vi "Laser Messenger.vi"(0 "Notifier Name":string, 2 "Action":T4, 5 "Emission On/Off":bool, 7 "Power (mW)":dbl, 11 "Laser Settings":T1, 13 "Exit While Busy (F)?":bool) -> (4 "Notifier Name Dup":string, 6 "Enabled (Interlock)?":bool, 8 "Light Emission?":bool, 10 "Laser Status":T3, 14 "Power (mW)":dbl, 15 "Laser Settings":T1)   [LabVIEW 2020]
uses:
  Laser Controls/Laser Actions.ctl
  Laser Controls/Laser Settings.ctl
  Laser Controls/Laser Parameters.ctl
  Laser Controls/Laser Status.ctl
  Laser Controls/Laser Notifier Element.ctl
panel:
  out "Error":errorcluster
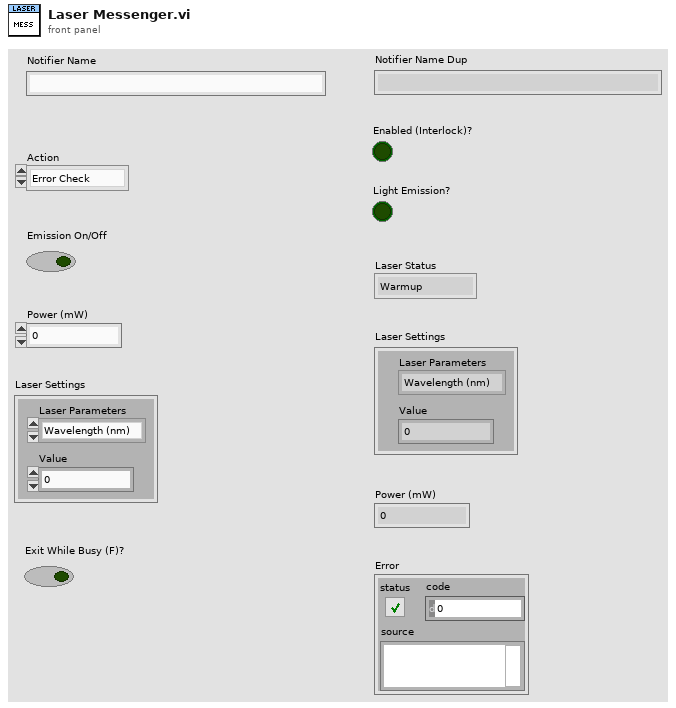
[diagram p1: front panel]
types:
  T1 = typedef "Laser Settings.ctl" = cluster{"Laser Parameters":T2, "Value":dbl}
  T2 = typedef "Laser Parameters.ctl" = enum16{"Wavelength (nm)", "Pulsing?", "Rep. Rate", "External Control"}
  T3 = typedef "Laser Status.ctl" = enum16{"Warmup", "Ready", "Emission", "Tuning", "Error"}
  T4 = typedef "Laser Actions.ctl" = enum16{"Error Check", "Set On/Off", "Set Power", "Set Parameter", "Get Power", "Get Status", "Get Parameter", "Quit"}
  T5 = typedef "Laser Notifier Element.ctl" = cluster{"Laser Action":T4, "Received?":bool, "Enabled (Interlock)?":bool, "Light Emission?":bool, "Power (mW)":dbl, "Settings":T1, "Status":T3, "Error":errorcluster}
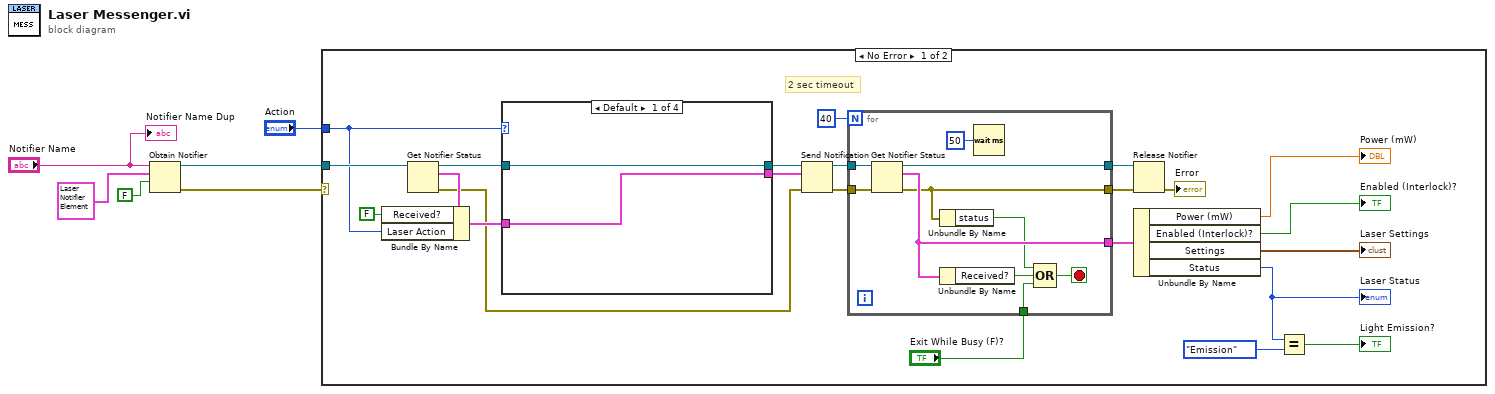
[diagram p0: block diagram]
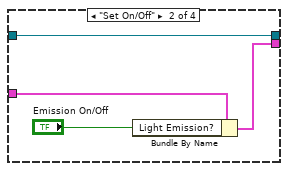
[diagram p2: hidden frame]
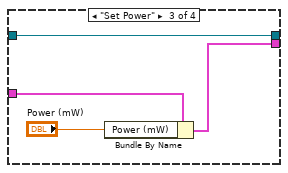
[diagram p3: hidden frame]
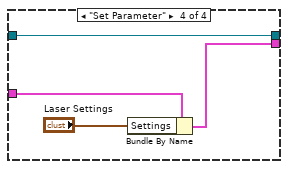
[diagram p4: hidden frame]
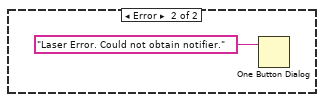
[diagram p5: hidden frame]
diagram:
  n1 = Obtain Notifier(name (unnamed)="Notifier Name", notification data type=T5 {"Laser Action"=enum."Set On/Off", "Received?"=FALSE, "Enabled (Interlock)?"=FALSE, "Light Emission?"=FALSE, "Power (mW)"=0.0, "Settings"={"Laser Parameters"=enum."Wavelength (nm)", "Value"=0.0}, "Status"=enum."Error", "Error"={"status"=FALSE, "code"=0, "source"=""}} ("Laser Notifier Element"), create if not found? (T)=FALSE) -> (notifier out=w2:refnum<notifier>, error out=w3:errorcluster)  [unwired: 1 in, 1 out]
  n2 = case shown="No Error" w3 {
    tunnel: w2 -> [w29 _]
    tunnel: "Action" -> [w24 _]
    frame No Error {
      # "2 sec timeout"
      n3 = Get Notifier Status(notifier=w29) -> (notifier out=w26:refnum<notifier>, current notification=w27:T5, error out=w12:errorcluster)  [unwired: 1 in, 2 out]
      n4 = Bundle By Name(cluster=w27, "Received?"=FALSE ("Running?"), "Laser Action"=w24) -> (w25:T5)
      n5 = case shown="Default" w24 {
        tunnel: w26 -> [w41 w44 w49 w50]
        tunnel: w25 -> [w40 w45 w48 w53]
        tunnel: [w41 w44 w49 w50] -> w18
        tunnel: [w40 w43 w46 w51] -> w17
        frame Default {
        }
        frame "Set On/Off" {
          n6 = Bundle By Name(cluster=w45, "Light Emission?"="Emission On/Off") -> (w43:T5)
        }
        frame "Set Power" {
          n7 = Bundle By Name(cluster=w48, "Power (mW)"="Power (mW)") -> (w46:T5)
        }
        frame "Set Parameter" {
          n8 = Bundle By Name(cluster=w53, "Settings"="Laser Settings") -> (w51:T5)
        }
      }
      n9 = Send Notification(notification=w17, notifier=w18, error in (no error)=w12) -> (notifier out=w16:refnum<notifier>, error out=w11:errorcluster)
      n10 = for {
        N: 40 -> [_]
        tunnel: w16 -> [w39]
        tunnel: "Exit While Busy (F)?" -> [w31]
        tunnel: w11 -> [w38]
        tunnel: [w34] -> w8
        tunnel: [w37] -> w9
        tunnel: [w36] -> w7
        stop <- w33 stop-if-true
        n11 = Get Notifier Status(notifier=w39, error in (no error)=w38) -> (notifier out=w37:refnum<notifier>, current notification=w36:T5, error out=w34:errorcluster)  [unwired: 2 out]
        n12 = Unbundle By Name(w34) -> ("status"=w30:bool)
        n13 = Unbundle By Name(w36) -> ("Received?"=w32:bool)
        n14 = Wait (ms)(milliseconds to wait=u32 50) -> ()  [unwired: 1 out]
        n15 = Compound Arithmetic op=OR(w30, w32, w31) -> (w33:bool)
      }
      n16 = Release Notifier(notifier=w9, error in (no error)=w8) -> (error out=→"Error":errorcluster)  [unwired: 1 in, 2 out]
      n17 = Unbundle By Name(w7) -> ("Power (mW)"=→"Power (mW)":dbl, "Enabled (Interlock)?"=→"Enabled (Interlock)?":bool, "Settings"=→"Laser Settings":T1, "Status"=w20:T3)
      "Laser Status" <- w20
      n18 = Equal?(x=w20, y=Laser_Status."Emission") -> (x = y?=→"Light Emission?":bool)
    }
    frame Error {
      n19 = One Button Dialog(message="Laser Error. Could not obtain notifier.") -> ()  [unwired: 1 in, 1 out]
    }
  }
  "Notifier Name Dup" <- "Notifier Name"
